vi "Send System Session.vi"(8 "error in":errorcluster, 11 "RT Management in":refnum<class "RT Management.lvclass">) -> (0 "error out":errorcluster, 2 "SysCfg Session":refnum<k21>, 3 "RT Management out":refnum<class "RT Management.lvclass">)   [LabVIEW 2016]
uses:
  RT Management.lvclass
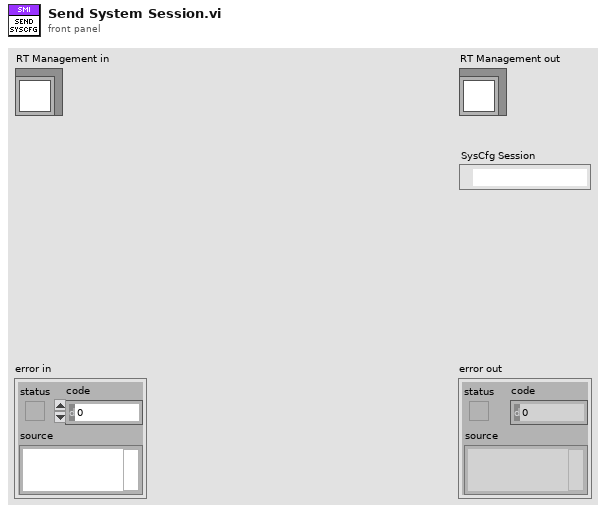
[diagram p1: front panel]
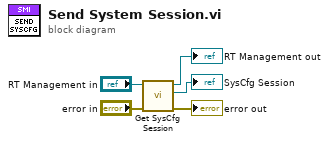
[diagram p0: block diagram]
diagram:
  n1 = call "Get SysCfg Session.vi"("error in (no error)"="error in", "RT Management Session in"="RT Management in") -> ("error out"=→"error out":errorcluster, "SysCfg Session"=→"SysCfg Session":refnum<k21>, "RT Management Session out"=→"RT Management out":refnum<class "RT Management.lvclass">)  [unwired: 7 in]
